vi "Configure Trigger (Pulse Width).vi"(0 "VISA resource name":refnum<visa-resource-name>, 1 "Pulse Width (1us)":dbl=1e-06, 2 "Trigger Pulse Mode (0: + Greater than)":u16(ring) items=["+ Greater Than", "+ Less Than", "+ Equal", "- Greater Than", "- Less Than", "- Equal"], 5 "Trigger Source (0: Channel 1)":i32(ring) items=["Channel 1"=0, "Channel 2"=1, "Channel 3"=2, "Channel 4"=3, "EXT"=4, "EXT5"=5, "Digital 0"=7, "Digital 1"=8, "Digital 2"=9, "Digital 3"=10, "Digital 4"=11, "Digital 5"=12, "Digital 6"=13, "Digital 7"=14, "Digital 8"=15, "Digital 9"=16, "Digital 10"=17, "Digital 11"=18, "Digital 12"=19, "Digital 13"=20, "Digital 14"=21, "Digital 15"=22], 7 "Trigger Level (0.0 V)":dbl, 11 "error in (no error)":errorcluster) -> (4 "VISA resource name out":refnum<visa-resource-name>, 15 "error out":errorcluster)   [LabVIEW 2012, in "RIGOL DS1000 Series.lvlib"]
doc: "Configures pulse width trigger settings for an oscilloscope."
uses:
  RIGOL DS1000 Series.lvlib
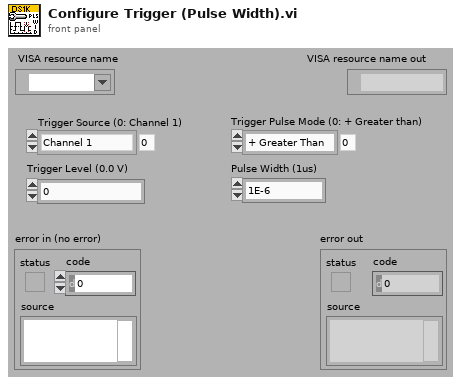
[diagram p1: front panel]
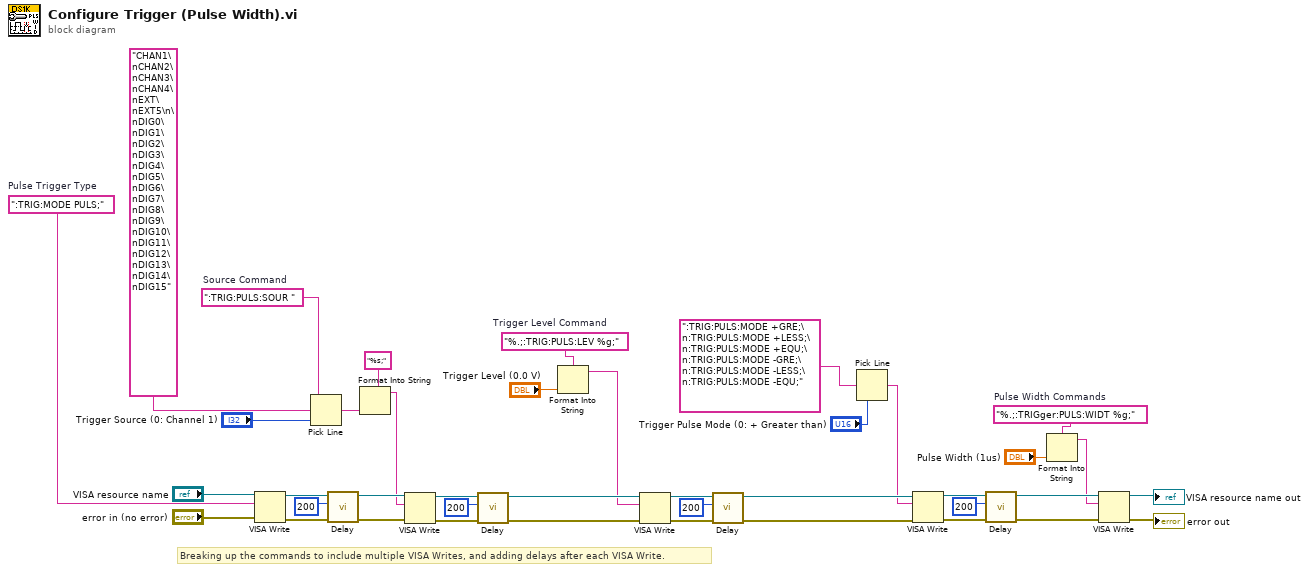
[diagram p0: block diagram]
diagram:
  w31 = "%.;:TRIG:PULS:LEV %g;"  # Trigger Level Command
  w2 = ":TRIG:MODE PULS;"  # Pulse Trigger Type
  w34 = ":TRIG:PULS:SOUR "  # Source Command
  w39 = "%.;:TRIGger:PULS:WIDT %g;"  # Pulse Width Commands
  # "Breaking up the commands to include multiple VISA Writes, and adding delays after each VISA Write."
  n1 = VISA Write(VISA resource name="VISA resource name", write buffer=w2, error in (no error)="error in (no error)") -> (VISA resource name out=w30:refnum<visa-resource-name>, error out=w29:errorcluster)  [unwired: 1 out]
  n2 = Pick Line(string ("")=w34, multi-line string="CHAN1\nCHAN2\nCHAN3\nCHAN4\nEXT\nEXT5\n\nDIG0\nDIG1\nDIG2\nDIG3\nDIG4\nDIG5\nDIG6\nDIG7\nDIG8\nDIG9\nDIG10\nDIG11\nDIG12\nDIG13\nDIG14\nDIG15" ("多行字符串"), line index="Trigger Source (0: Channel 1)") -> (output string=w36:string)
  n3 = call "Delay.vi"("error in (no error)"=w29, "Delay (ms)"=u32 200, "VISA resource name"=w30) -> ("error out"=w21:errorcluster, "VISA resource name out"=w22:refnum<visa-resource-name>)  [unwired: 7 out]
  n4 = Format Into String(format string="%s;", w36) -> (resulting string=w20:string)  [unwired: 2 in, 1 out]
  n5 = VISA Write(VISA resource name=w22, write buffer=w20, error in (no error)=w21) -> (VISA resource name out=w25:refnum<visa-resource-name>, error out=w24:errorcluster)  [unwired: 1 out]
  n6 = call "Delay.vi"("error in (no error)"=w24, "Delay (ms)"=u32 200, "VISA resource name"=w25) -> ("error out"=w15:errorcluster, "VISA resource name out"=w16:refnum<visa-resource-name>)  [unwired: 7 out]
  n7 = Format Into String(format string=w31, "Trigger Level (0.0 V)") -> (resulting string=w14:string)  [unwired: 2 in, 1 out]
  n8 = VISA Write(VISA resource name=w16, write buffer=w14, error in (no error)=w15) -> (VISA resource name out=w19:refnum<visa-resource-name>, error out=w18:errorcluster)  [unwired: 1 out]
  n9 = call "Delay.vi"("error in (no error)"=w18, "Delay (ms)"=u32 200, "VISA resource name"=w19) -> ("error out"=w9:errorcluster, "VISA resource name out"=w10:refnum<visa-resource-name>)  [unwired: 7 out]
  n10 = Pick Line(multi-line string=":TRIG:PULS:MODE +GRE;\n:TRIG:PULS:MODE +LESS;\n:TRIG:PULS:MODE +EQU;\n:TRIG:PULS:MODE -GRE;\n:TRIG:PULS:MODE -LESS;\n:TRIG:PULS:MODE -EQU;", line index="Trigger Pulse Mode (0: + Greater than)") -> (output string=w8:string)  [unwired: 1 out]
  n11 = VISA Write(VISA resource name=w10, write buffer=w8, error in (no error)=w9) -> (VISA resource name out=w13:refnum<visa-resource-name>, error out=w12:errorcluster)  [unwired: 1 out]
  n12 = call "Delay.vi"("error in (no error)"=w12, "Delay (ms)"=u32 200, "VISA resource name"=w13) -> ("error out"=w6:errorcluster, "VISA resource name out"=w7:refnum<visa-resource-name>)  [unwired: 7 out]
  n13 = Format Into String(format string=w39, "Pulse Width (1us)") -> (resulting string=w5:string)  [unwired: 2 in, 1 out]
  n14 = VISA Write(VISA resource name=w7, write buffer=w5, error in (no error)=w6) -> (VISA resource name out=→"VISA resource name out":refnum<visa-resource-name>, error out=→"error out":errorcluster)  [unwired: 1 out]
